vi "Generate Two Random Indices In Ascending Order.vi"(11 "Schedule":u16[](array[numeric])) -> (2 "Index 2":i32, 3 "Index 1":i32)   [LabVIEW 2013, in "GA.lvclass"]
uses:
  GA.lvclass
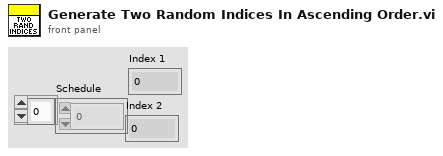
[diagram p1: front panel]
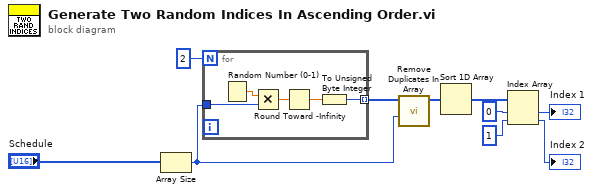
[diagram p0: block diagram]
diagram:
  n1 = Array Size(array="Schedule") -> (size(s)=w3:i32)
  n2 = for {
    N: 2 -> [_]
    tunnel: w3 -> [w14]
    tunnel: [w11] -> w8 mode=indexing
    n3 = Random Number (0-1)() -> (number: 0 to 1=w15:dbl)
    n4 = Multiply(x=w15, y=w14) -> (x*y=w13:dbl)
    n5 = Round Toward -Infinity(1:w13) -> (0:w12:dbl)
    n6 = To Unsigned Byte Integer(number=w12) -> (unsigned 8bit integer=w11:u8)
  }
  n7 = call "Remove Duplicates In Array.vi"("Max Index Bound"=w3, "Random Numbers Array"=w8) -> ("Random Numbers Array without Duplicates"=w7:i32[])  [unwired: 9 in]
  n8 = Sort 1D Array(array=w7) -> (sorted array=w6:i32[])
  n9 = Index Array(array=w6, index #1=0 ("index"), index #2=1 ("index")) -> (element #1=→"Index 1":i32, element #2=→"Index 2":i32)
